vi "Transfer_Img_To_1D_Rev_Arr.vi"(8 "error in":errorcluster, 11 "[IN] Original Image":T1) -> (0 "error out":errorcluster, 2 "[OUT] Threshold Initial":u16, 3 "[OUT] 1D Sort Rever Img":u16[](array[numeric]))   [LabVIEW 2020]
doc: "Draws the cross for showing a center of mass"
uses:
  <vilib>/vision/Image Controls.llb/IMAQ Image.ctl
  <vilib>/vision/NI_Vision_Development_Module.lvlib
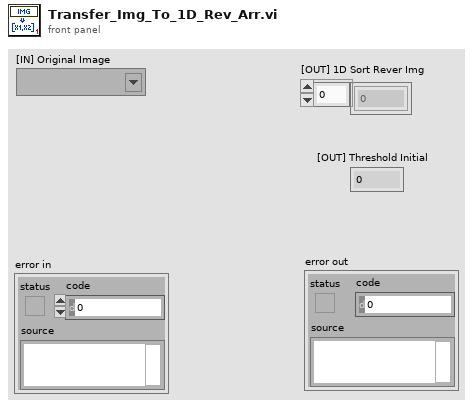
[diagram p1: front panel]
types:
  T1 = typedef "IMAQ Image.ctl" = refnum<image>
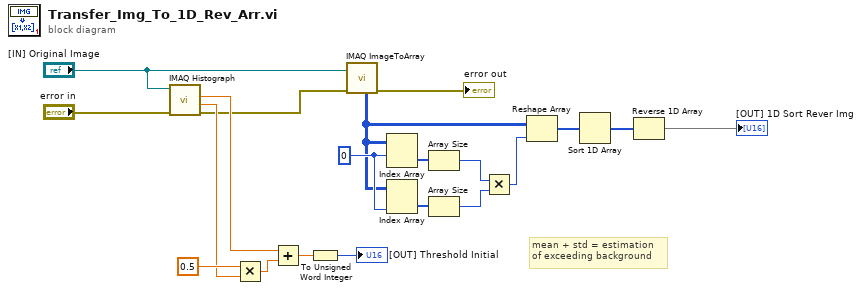
[diagram p0: block diagram]
diagram:
  w13 = 0 ("index (row)")
  # "mean + std = estimation\nof exceeding background"
  n1 = call "IMAQ Histograph"("error in (no error)"="error in", "Image"="[IN] Original Image") -> ("error out"=w6:errorcluster, "Standard  Deviation"=w15:sgl, "Mean Value"=w16:sgl)  [unwired: 6 in, 1 out]
  n2 = Multiply(x=sgl 0.5, y=w15) -> (x*y=w17:sgl)
  n3 = Add(x=w16, y=w17) -> (x+y=w19:sgl)
  n4 = To Unsigned Word Integer(number=w19) -> (unsigned 16bit integer=→"[OUT] Threshold Initial":u16)
  n5 = call "IMAQ ImageToArray"("error in (no error)"=w6, "Image"="[IN] Original Image") -> ("Image Pixels (U16)"=w10:u16[][], "error out"=→"error out":errorcluster)  [unwired: 2 in, 3 out]
  n6 = Index Array(array=w10, index (row)=w13) -> (element=w12:u16[])  [unwired: 1 in]
  n7 = Index Array(array=w10, index (col)=w13) -> (element=w11:u16[])  [unwired: 1 in]
  n8 = Array Size(array=w12) -> (size(s)=w8:i32)
  n9 = Array Size(array=w11) -> (size(s)=w7:i32)
  n10 = Multiply(x=w8, y=w7) -> (x*y=w9:i32)
  n11 = Reshape Array(w10, w9) -> (w3:u16[])
  n12 = Sort 1D Array(array=w3) -> (sorted array=w4:u16[])
  n13 = Reverse 1D Array(array=w4) -> (reversed array=→"[OUT] 1D Sort Rever Img":u16[])
